vi "XIPIN_AXI_Bus_Functional_Model_2_1.vi"   [LabVIEW 2017]
doc: "The AXI Bus Functional Model (BFM) solution, created for Xilinx by Cadence Design Systems, enables Xilinx customers to verify and simulate communication with AXI-based IP that is being developed. Complete verification of these interfaces and protocol compliance is outside the scope of the AXI BFM solution; for compliance testing and complete system-level verification of AXI interfaces, the Cadence AXI UVC can be used.\n\nThe AXI BFM IP delivers example test benches and example scripts that demonstrate the use of the BFM Test Writing APIs for AXI3, AXI4, AXI4-Lite, and AXI4-Stream masters and slaves.\n\nThe AXI BFM solution is an optional product that is purchased separate from the ISE software. Licensing is handled through the standard Xilinx licensing scheme. A new license feature, XILINX_AXI_BFM, is needed in addition to the standard ISE license\nfeatures. A license is checked out at simulation run time. While the Xilinx ISE software does not need to be running while the AXI BFM solution is in use, the AXI BFM will only operate on a computer that has the Xilinx software installed and licensed.\n------------------------------------\n<b>Need License</b> : No"
uses:
  <vilib>/rvi/XilinxIP/XIPIN_XNode/niFpgaXIPIN.xnode
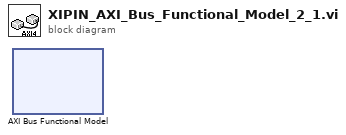
[diagram p0: block diagram]
diagram:
  n1 = xnode ("AXI Bus Functional Model")() -> ()
